vi "Mask Calculations.vi"(8 "Any Targets":bool, 10 "Index of Top Rectangle":i32, 11 "Scored Particle Info":T2(array[cluster])) -> (0 "Vertical Center of Rectangle":dbl, 1 "Valid Target":bool, 2 "Horizontal Center of Rectangle":dbl, 3 "Cluster":T1)   [LabVIEW 2013]
panel:
  out "Array":dbl[](array[numeric])
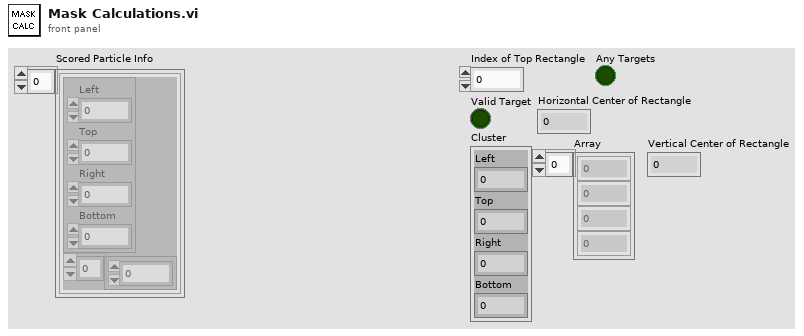
[diagram p1: front panel]
types:
  T1 = cluster{"Left":dbl, "Top":dbl, "Right":dbl, "Bottom":dbl}
  T2 = cluster{cluster{"Left":dbl, "Top":dbl, "Right":dbl, "Bottom":dbl}, dbl[]}[]
  T3 = cluster{cluster{"Left":dbl, "Top":dbl, "Right":dbl, "Bottom":dbl}, dbl[]}
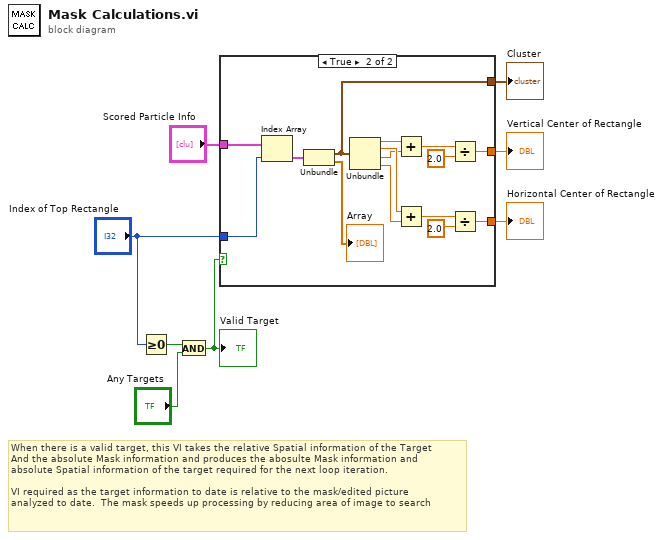
[diagram p0: block diagram]
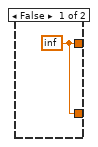
[diagram p2: hidden frame]
diagram:
  # "When there is a valid target, this VI takes the relative Spatial information of the Target\nAnd the absolute Mask information and produces the abosulte Mask information and \nabsolute Spatial information of the target required for the next loop iteration.\n\nVI required as the target information to date is relative to the mask/edited picture\nanalyzed to date.  The mask speeds up processing by reducing area of image to search"
  n1 = Greater Or Equal To 0?(x="Index of Top Rectangle") -> (x >= 0?=w5:bool)
  n2 = And(x=w5, y="Any Targets") -> (x .and. y?=w3:bool)
  "Valid Target" <- w3
  n3 = case shown="True" w3 {
    tunnel: "Scored Particle Info" -> [_ w24]
    tunnel: [w9 w23] -> w7
    tunnel: "Index of Top Rectangle" -> [_ w17]
    tunnel: [w9 w12] -> w2
    tunnel: [_ w11] -> w1
    frame False {
      w9 = inf
    }
    frame True {
      n4 = Index Array(array=w24, index=w17) -> (element=w18:T3)
      n5 = Unbundle(w18) -> (w11:T1, →"Array":dbl[])
      n6 = Unbundle(w11) -> ("Left"=w16:dbl, "Top"=w20:dbl, "Right"=w15:dbl, "Bottom"=w19:dbl)
      n7 = Add(x=w16, y=w15) -> (x+y=w14:dbl)
      n8 = Add(x=w20, y=w19) -> (x+y=w21:dbl)
      n9 = Divide(x=w14, y=2.0) -> (x/y=w12:dbl)
      n10 = Divide(x=w21, y=2.0) -> (x/y=w23:dbl)
    }
  }
  "Horizontal Center of Rectangle" <- w7
  "Vertical Center of Rectangle" <- w2
  "Cluster" <- w1
